vi "Read Charact Standard List.vi"(8 "error in (no error)":errorcluster, 11 "Vector Abstract Path Group in":refnum<class "Vector Abstract Path Group.lvclass">) -> (0 "error out":errorcluster, 2 "Charact Standard List":T1[](array[typedef]), 3 "Vector Abstract Path Group out":refnum<class "Vector Abstract Path Group.lvclass">)   [LabVIEW 2023, in "RFFixtureCharact.Public.lvlib" / "Vector Abstract Path Group.lvclass"]
uses:
  Vector Abstract Path Group.lvclass
  Vector Abstract Path Group.lvclass/Vector Abstract Path Group.ctl
  Instruments/Cal Standard/Type Definitions/Standard Type.ctl
  Instruments/RFFixtureCharact.Instruments.lvlib
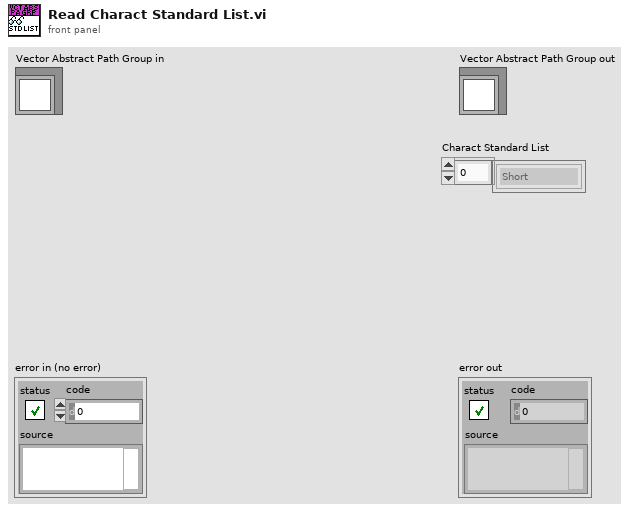
[diagram p1: front panel]
types:
  T1 = typedef "RFFixtureCharact.Instruments.lvlib/Standard Type.ctl" = enum16{"Short", "Open", "Load", "PowerMeter", "None"}
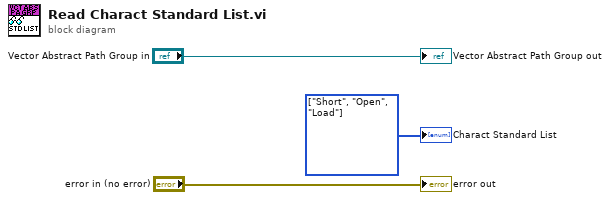
[diagram p0: block diagram]
diagram:
  w1 = T1[] [enum."Short", enum."Open", enum."Load"] items=["Short", "Open", "Load", "PowerMeter", "None"] ("Charact Standard List")
  "error out" <- "error in (no error)"
  "Vector Abstract Path Group out" <- "Vector Abstract Path Group in"
  "Charact Standard List" <- w1
